vi "Export Waveform Graph Image to Notebook.vi"(8 "Error In":errorcluster, 9 "Multiwaveform Graph Refnum":refnum<vi>, 11 "Notebook Q":refnum<queue>) -> (0 "Error Out":errorcluster)   [LabVIEW 2021, in "Notebook.lvlib"]
uses:
  Notebook.lvlib
  Notebook Action Q Element.ctl
  Notebook Action List.ctl
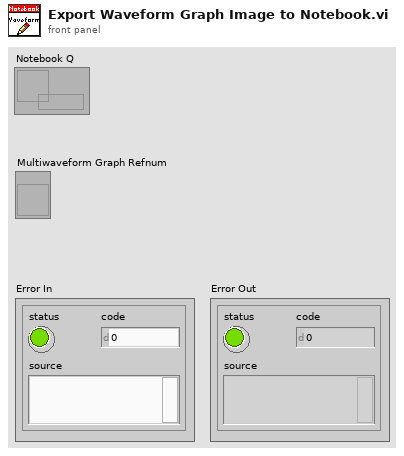
[diagram p1: front panel]
types:
  T1 = typedef "Notebook.lvlib/Notebook Action Q Element.ctl" = cluster{"Action":T2, "Variant":variant}
  T2 = typedef "Notebook.lvlib/Notebook Action List.ctl" = enum16{"Idle", "Init", "Check Content Change", "User added content", "Program added text", "Program added Picture ", "Save Notebook", "Quit", "Open", "Close", "Update Window Title"}
  T3 = typedef "imagedata.ctl" = cluster{"image type":i32, "image depth":i32, "image":u8[], "mask":u8[], "colors":u32[], "Rectangle":cluster{"left":i16, "top":i16, "right":i16, "bottom":i16}}
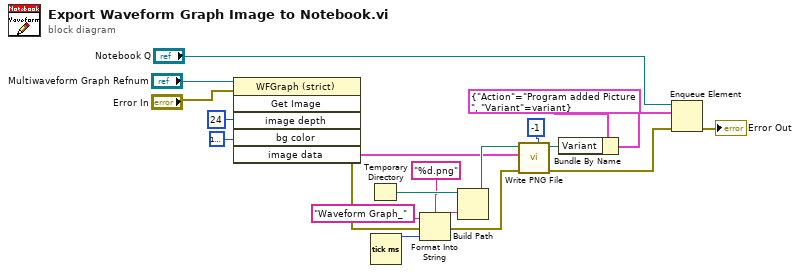
[diagram p0: block diagram]
diagram:
  n1 = invoke on="Invoke Node" class="WFGraph (strict)" method="Get Image"(reference="Multiwaveform Graph Refnum", error in="Error In", "image depth"=24 ("Image Depth"), "bg color"=u32 16777226) -> (error out=w2:errorcluster, "image data"=w9:T3)  [unwired: 2 in, 4 out]
  n2 = Temporary Directory() -> (w15:path)
  n3 = Tick Count (ms)() -> (millisecond timer value=w14:u32)
  n4 = Format Into String(format string="%d.png", initial string="Waveform Graph_", error in=w2, w14) -> (resulting string=w13:string, error out=w1:errorcluster)
  n5 = Build Path(base path=w15, name or relative path=w13) -> (appended path=w10:path)
  n6 = call <vilib>:"Write PNG File.vi"("compression (default)"=-1, "error in (no error)"=w1, "image data"=w9, "path to PNG file"=w10) -> ("error out"=w4:errorcluster, "path"=w8:path)  [unwired: 6 in]
  n7 = Bundle By Name(cluster=T1 {"Action"=enum."Program added Picture ", "Variant"=variant} ("element"), "Variant"=w8) -> (w6:T1)
  n8 = Enqueue Element(queue="Notebook Q", element=w6, error in (no error)=w4) -> (error out=→"Error Out":errorcluster)  [unwired: 1 in, 2 out]
